vi "GetButtonRefs.vi"(11 "BtnRefs":T1) -> (3 "BtnRefs":T1)   [LabVIEW 2014, in "Framework.lvlib"]
uses:
  Framework.lvlib
  TypeDefs/clFrontPanelButtonRefs.ctl
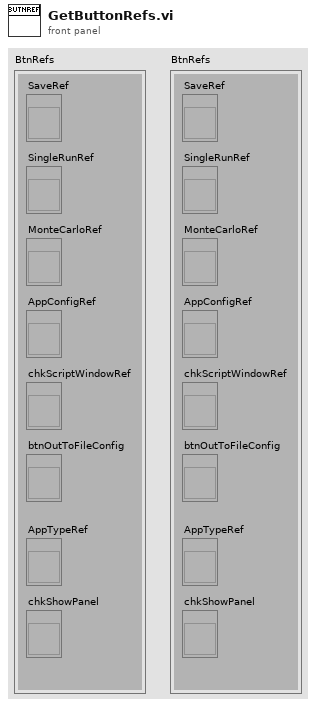
[diagram p1: front panel]
types:
  T1 = typedef "Framework.lvlib/clFrontPanelButtonRefs.ctl" = cluster{"SaveRef":refnum<vi>, "SingleRunRef":refnum<vi>, "MonteCarloRef":refnum<vi>, "AppConfigRef":refnum<vi>, "chkScriptWindowRef":refnum<vi>, "btnOutToFileConfig":refnum<vi>, "AppTypeRef":refnum<vi>, "chkShowPanel":refnum<vi>}
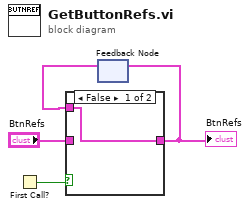
[diagram p0: block diagram]
diagram:
  n1 = First Call?() -> (First Call?: T/F=w4:bool)
  n2 = feedback #1() -> (w2:T1)  [unwired: 1 in]
  n3 = case shown="False" w4 {
    tunnel: [w5 w6] -> w1
    tunnel: "BtnRefs" -> [_ w6]
    tunnel: w2 -> [w5 _]
    frame False {
    }
    frame True {
    }
  }
  "BtnRefs" <- w1
  n4 = feedback-in #1(w1) -> ()
